vi "Drive Controller.vi"(8 "error in":errorcluster) -> ()   [LabVIEW 2018]
doc: "This VI executes continuously carrying out the current operation and responding to updates or new operation requests. It will often contain the timing or control code that is difficult to place directly in TeleOp. This VI generally opens all sensors and motors and isolates the rest of the robot code from knowing implementation details of how the operations are carried out."
uses:
  <vilib>/Rock Robotics/WPI/Framework/Completion Status.ctl
  Drive Setpoints.ctl
  Drive Operations.ctl
  <vilib>/Rock Robotics/WPI/SafetyOutput/WPI_SafetyOutputConfigMenu.ctl
  <vilib>/Rock Robotics/WPI/Utilities/WPI_GetSetVariantRefNum.vi
  <vilib>/Rock Robotics/SystemInterfaces/DIO/FPGA_DIOPWMChannel.ctl
  <vilib>/Rock Robotics/WPI/RobotDrive/WPI_RobotDriveOpen4MotorWithTalonSRX.vi
panel:
  in  "Interactive Values":T1
  in  "Buttons":cluster{"Execute Cmd":bool, "Abort Cmd":bool}
  out "Command Timing":cluster{"Start Time (ms)":u32, "Iterations":i32}
  out "Status":T3
  out "Setpoints":T4(graph)
  out "Current\nCmd":string
  # "Tip: The graph shows the motor setpoints. It may also be helpful to observe inputs and sensor values.\nYou may also want to display tuning or debugging controls."
  # "Interactive Command: You may fill in the settings for a command\nand schedule it with the Execute button. You can observe and abort\nany command while fine tuning the code for the controller."
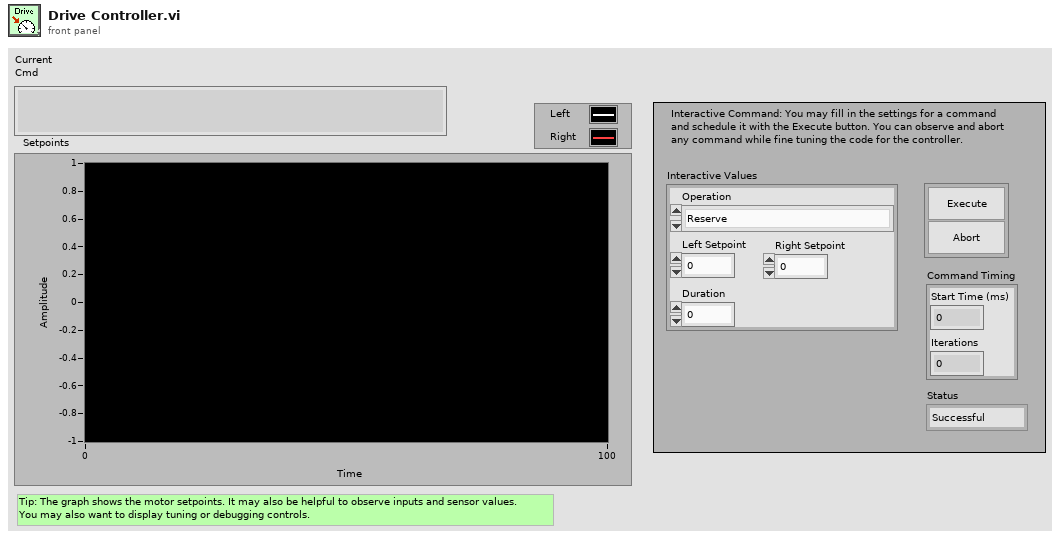
[diagram p1: front panel]
types:
  T1 = typedef "Drive Setpoints.ctl" = cluster{"Operation":T2, "Left Setpoint":dbl, "Right Setpoint":dbl, "Duration":dbl}
  T2 = typedef "Drive Operations.ctl" = enum16{"Reserve", "Read Current", "Immediate", "Drive for Time", "Drive for Distance"}
  T3 = typedef "Completion Status.ctl" = enum16{"Successful", "Aborted", "Incomplete"}
  T4 = cluster{"Left Setpoint":dbl, "Right Setpoint":dbl}
  T5 = typedef "WPI_SafetyOutputConfigMenu.ctl" = enum16{"Enable", "Disable"}
  T6 = typedef "FPGA_DIOPWMChannel.ctl" = enum8{"PWM 0", "PWM 1", "PWM 2", "PWM 3", "PWM 4", "PWM 5", "PWM 6", "PWM 7", "PWM 8", "PWM 9", "PWM MXP 0", "PWM MXP 1", "PWM MXP 2", "PWM MXP 3", "PWM MXP 4", "PWM MXP 5", "PWM MXP 6", "PWM MXP 7", "PWM MXP 8", "PWM MXP 9", "Invalid"}
  T7 = typedef "WPI_RobotDriveDevRef.ctl" = cluster{"DevStatus":errorcluster, "Motors[]":T8[], "Square Inputs":bool, "Max Output":dbl}
  T8 = typedef "WPI_MotorControlDeviceRef.ctl" = cluster{"DeviceStatus":errorcluster, "Type":T9, "PWM":cluster{"PWM Channel":T6, "DeadBand":T10}, "CAN":cluster{"Device Number":u8, "SetOutput VI Ref":variant, "GetOutput VI Ref":variant, "Enable VI Ref":variant, "Disable VI Ref":variant, "Data":variant}, "Invert":bool, "DIO PWM":cluster{"PWM \"Enable\" Channel":T6, "DIOChannel":T11, "PWM Rate":dbl}}
  T9 = typedef "WPI_MotorControlType.ctl" = enum16{"PWM", "CAN", "DIO PWM"}
  T10 = typedef "WPI_PWMDeadband.ctl" = cluster{"Name":string, "maxPositivePwm":i32, "minPositivePwm":i32, "centerPwm":i32, "maxNegativePwm":i32, "minNegativePwm":i32, "angularRange":u16}
  T11 = typedef "FPGA_DIOChannel.ctl" = enum8{"DIO 0", "DIO 1", "DIO 2", "DIO 3", "DIO 4", "DIO 5", "DIO 6", "DIO 7", "DIO 8", "DIO 9", "DIO MXP 0", "DIO MXP 1", "DIO MXP 2", "DIO MXP 3", "DIO MXP 4", "DIO MXP 5", "DIO MXP 6", "DIO MXP 7", "DIO MXP 8", "DIO MXP 9", "DIO MXP 10", "DIO MXP 11", "DIO MXP 12", "DIO MXP 13", "DIO MXP 14", "DIO MXP 15", "SPI Port CS1", "SPI Port CS2", "SPI Port CS3", "SPI Port MISO", "SPI Port MOSI", "Invalid"}
  T12 = typedef "Command Status Info.ctl" = cluster{"Name":string, "Status":T3, "notifier out":T13}
  T13 = typedef "Completion Notifier.ctl" = refnum<notifier>
  T14 = cluster{"SubSystem Data":T1, cluster{"Start Time (ms)":u32, "Iterations":i32}, cluster{"Command Info":T12, "Description":string, "Default Command":T1, "queue out":refnum<queue>, "Subsystem Name":string}}
  T15 = cluster{"SubSystem Data":T1, cluster{"Start Time (ms)":u32, "Iterations":i32}, "Default Command Arguments":cluster{"Command Info":T12, "Description":string, "Default Command":T1, "queue out":refnum<queue>, "Subsystem Name":string}}
  T16 = cluster{"Don't move motors while reserved":dbl, "Don't move motors while reserved":dbl}
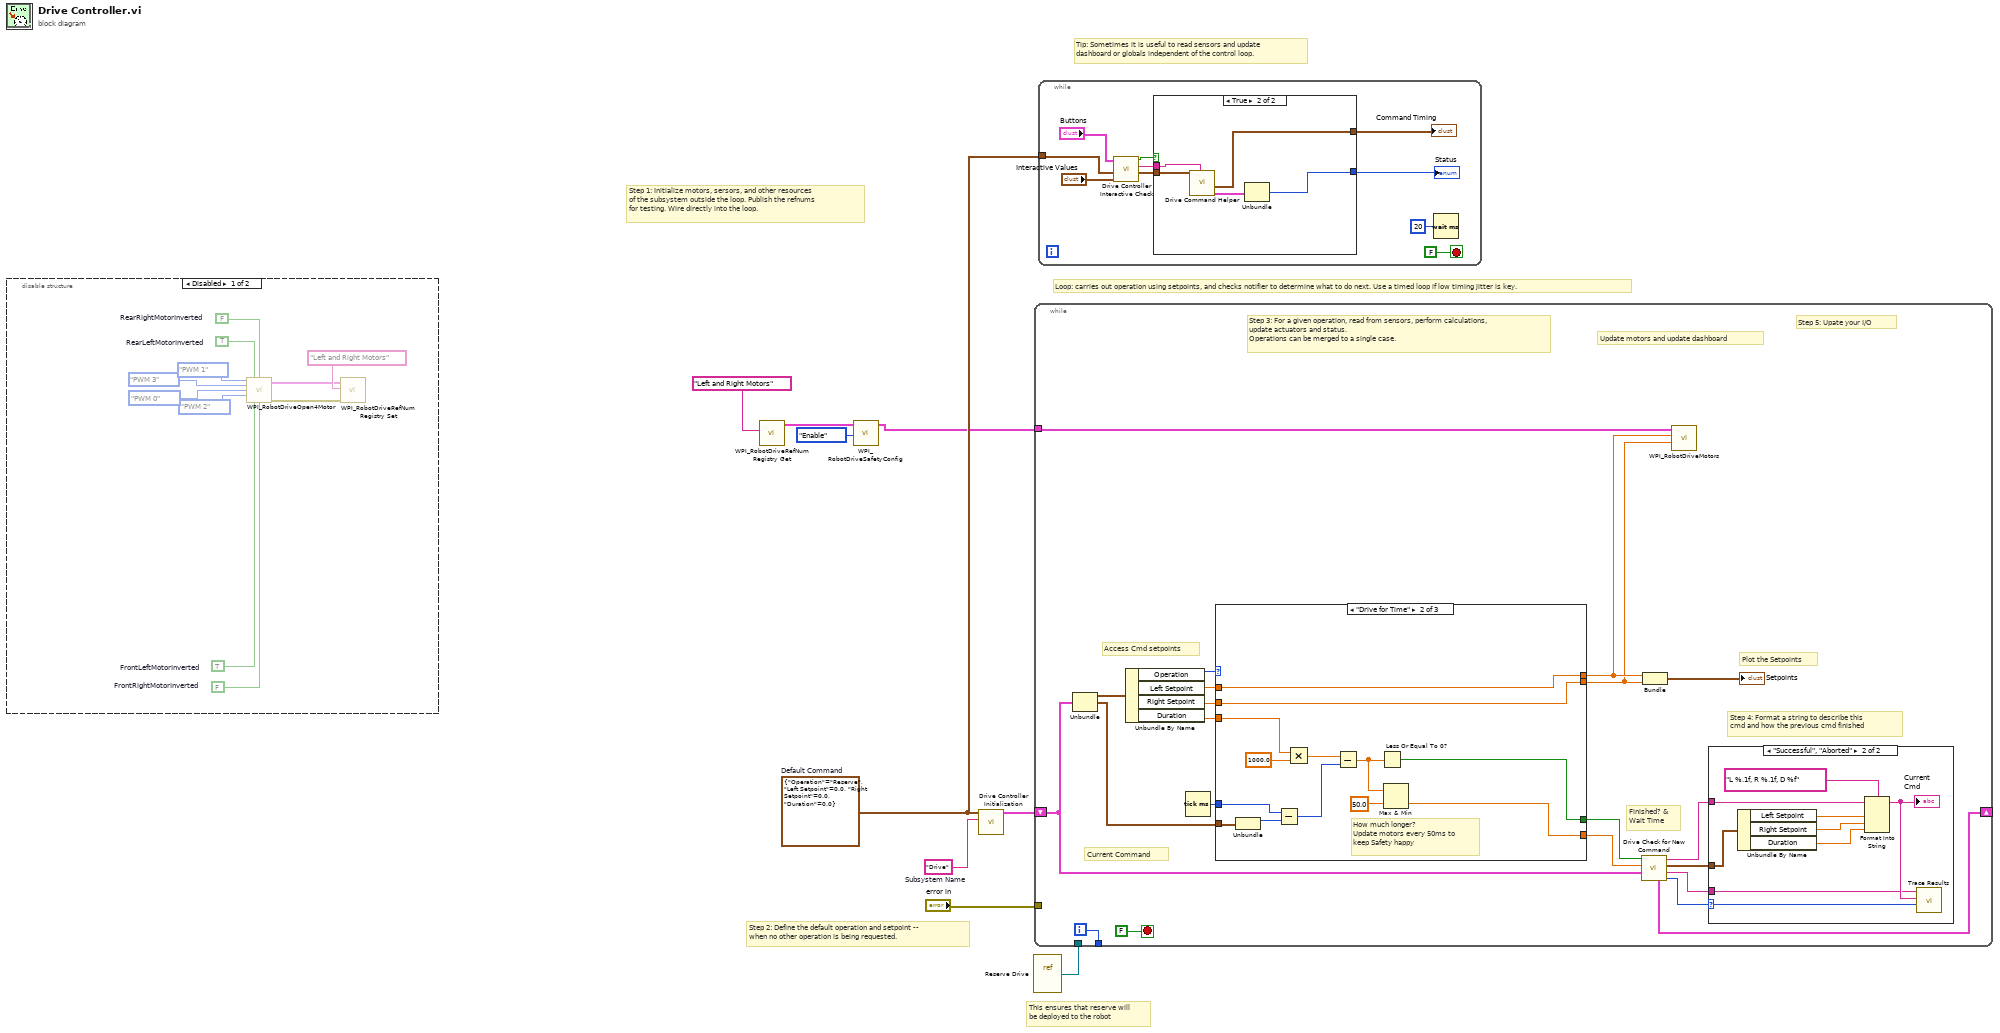
[diagram p0: block diagram]
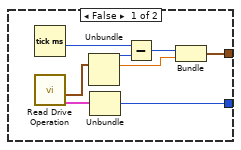
[diagram p3: hidden frame]
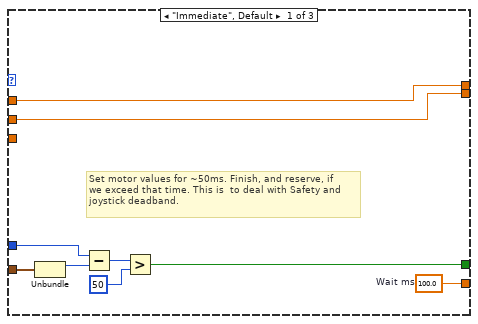
[diagram p5: hidden frame]
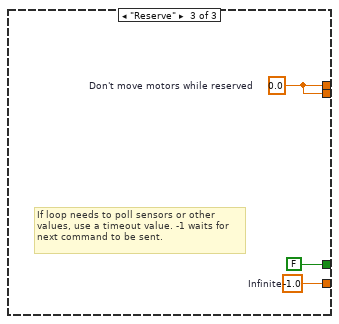
[diagram p6: hidden frame]
diagram:
  w5 = T1 {"Operation"=enum."Reserve", "Left Setpoint"=0.0, "Right Setpoint"=0.0, "Duration"=0.0}  # Default Command
  w9 = "Drive"  # Subsystem Name
  # "This ensures that reserve will\nbe deployed to the robot"
  # "Tip: Sometimes it is useful to read sensors and update\ndashboard or globals independent of the control loop."
  # "Step 2: Define the default operation and setpoint --\nwhen no other operation is being requested."
  # "Step 1: Initialize motors, sersors, and other resources\nof the subsystem outside the loop. Publish the refnums\nfor testing. Wire directly into the loop."
  # "Loop: carries out operation using setpoints, and checks notifier to determine what to do next. Use a timed loop if low timing jitter is key."
  n1 = disable-structure shown="Disabled" {
    frame Disabled {
      w19 = TRUE  # FrontLeftMotorInverted
      w16 = FALSE  # FrontRightMotorInverted
      w18 = TRUE  # RearLeftMotorInverted
      w17 = FALSE  # RearRightMotorInverted
      n2 = call-poly <vilib>:"WPI_RobotDriveOpen4Motor.vi"("Rear Left Motor"=FPGA_DIOPWMChannel."PWM 1" ("Rear Right Motor"), "Rear Left Motor Inverted"=w18, "Rear Right Motor Inverted"=w17, "Rear Right Motor"=FPGA_DIOPWMChannel."PWM 3" ("Front Left Motor"), "Front Left Motor"=FPGA_DIOPWMChannel."PWM 0" ("Rear Left Motor"), "Front Right Motor"=FPGA_DIOPWMChannel."PWM 2", "Front Left Motor Inverted"=w19, "Front Right Motor Inverted"=w16) -> ("RobotDriveDevRef"=w12:T7, "error out"=w11:errorcluster)  [unwired: 6 in]
      n3 = call <vilib>:"WPI_RobotDriveRefNum Registry Set.vi"("error in (no error)"=w11, "refnum name"="Left and Right Motors", "RobotDriveDevRef"=w12) -> ()  [unwired: 1 in, 8 out]
    }
    frame Enabled {
    }
  }
  n4 = call <vilib>:"WPI_RobotDriveRefNum Registry Get.vi"("refnum name"="Left and Right Motors") -> ("RobotDriveDevRef"=w4:T7)  [unwired: 9 in, 1 out]
  n5 = call <vilib>:"WPI_RobotDriveSafetyConfig.vi"("mode"=WPI_SafetyOutputConfigMenu."Enable", "RobotDriveDevRef"=w4) -> ("RobotDriveDevRef"=w1:T7)  [unwired: 8 in, 1 out]
  n6 = call "Drive Controller Initialization.vi"("Subsystem Name"=w9, "Default Command"=w5) -> ("Current Command"=w7:T14)  [unwired: 9 in]
  n7 = vi-ref "Reserve Drive.vi"() -> (w6:refnum<vi>)
  n8 = while {
    shift-right: [w31] -> _
    shift-left: w7 -> [w24]
    tunnel: [w40] -> _
    tunnel: "error in" -> [_]
    tunnel: w6 -> [_]
    tunnel: w1 -> [w23]
    i -> [w40]
    stop <- FALSE stop-if-true
    # "Step 5: Upate your I/O"
    # "Step 4: Format a string to describe this\ncmd and how the previous cmd finished"
    # "Current Command"
    # "Update motors and update dashboard"
    # "Plot the Setpoints"
    # "Access Cmd setpoints"
    # "Finished? &\nWait Time"
    # "Step 3: For a given operation, read from sensors, perform calculations,\nupdate actuators and status.\nOperations can be merged to a single case."
    n9 = Unbundle(w24) -> ("SubSystem Data"=w38:T1, w25:cluster{"Start Time (ms)":u32, "Iterations":i32})  [unwired: 1 out]
    n10 = Unbundle By Name(w38) -> ("Operation"=w37:T2, "Left Setpoint"=w36:dbl, "Right Setpoint"=w35:dbl, "Duration"=w34:dbl)
    n11 = Tick Count (ms)() -> (millisecond timer value=w33:u32)
    n12 = case shown="\"Drive for Time\"" w37 {
      tunnel: [w59 w60 w75] -> w30
      tunnel: [w52 w67 FALSE ("ignore previous (F)")] -> w29
      tunnel: w25 -> [w51 w69 _]
      tunnel: [w58 w66 w73] -> w22
      tunnel: [w57 w65 w73] -> w21
      tunnel: w36 -> [w58 w66 _]
      tunnel: w35 -> [w57 w65 _]
      tunnel: w34 -> [_ w64 _]
      tunnel: w33 -> [w53 w63 _]
      frame "Immediate", Default {
        w59 = 100.0  # Wait ms
        # "Set motor values for ~50ms. Finish, and reserve, if\nwe exceed that time. This is  to deal with Safety and\njoystick deadband."
        n13 = Unbundle(w51) -> ("Start Time (ms)"=w54:u32)  [unwired: 1 out]
        n14 = Subtract(x=w53, y=w54) -> (x-y=w55:u32)
        n15 = Greater?(x=w55, y=u8 50 ("Left Motor")) -> (0:w52:bool)
      }
      frame "Drive for Time" {
        # "How much longer?\nUpdate motors every 50ms to\nkeep Safety happy"
        n16 = Unbundle(w69) -> ("Start Time (ms)"=w68:u32)  [unwired: 1 out]
        n17 = Subtract(x=w63, y=w68) -> (x-y=w72:u32)
        n18 = Multiply(x=w64, y=1000.0) -> (x*y=w71:dbl)
        n19 = Subtract(x=w71, y=w72) -> (x-y=w62:dbl)
        n20 = Less Or Equal To 0?(x=w62) -> (x <= 0?=w67:bool)
        n21 = Max & Min(x=w62, y=50.0) -> (min(x,y)=w60:dbl)  [unwired: 1 out]
      }
      frame "Reserve" {
        w73 = 0.0  # Don't move motors while reserved
        w75 = -1.0  # Infinite
        # "If loop needs to poll sensors or other\nvalues, use a timeout value. -1 waits for\nnext command to be sent."
      }
    }
    n22 = call "Drive Check for New Command.vi"("input cluster"=w24, "Wait time (ms)"=w30, "Finished?"=w29) -> ("Completion"=w32:T3, "Subsystem Name"=w26:string, "Current Command"=w27:T1, "Initial Trace String"=w28:string, "Next Command"=w31:T15)  [unwired: 4 in]
    n23 = Bundle("Don't move motors while reserved"=w22, "Don't move motors while reserved"=w21) -> (→"Setpoints":T16)  [unwired: 1 in]
    n24 = call <vilib>:"WPI_RobotDriveMotors.vi"("RightSpeed"=w21, "LeftSpeed"=w22, "RobotDriveDevRef"=w23) -> ()  [unwired: 6 in, 3 out]
    n25 = case shown="\"Successful\", \"Aborted\"" w32 {
      selector: w32 -> [_ w50]
      tunnel: w28 -> [_ w45]
      tunnel: w27 -> [_ w46]
      tunnel: w26 -> [_ w42]
      frame "Incomplete", Default {
        # "Continuing current command"
      }
      frame "Successful", "Aborted" {
        # "Report and setup for next command"
        n26 = Unbundle By Name(w46) -> ("Left Setpoint"=w48:dbl, "Right Setpoint"=w49:dbl, "Duration"=w43:dbl)
        n27 = Format Into String(format string="L %.1f, R %.1f, D %f", initial string=w45, w48, w49, w43) -> (resulting string=w44:string)  [unwired: 1 in, 1 out]
        "Current\nCmd" <- w44
        n28 = call <vilib>:"Trace Results.vi"("Status of previous command"=w50, "Description"=w44, "Subsystem"=w42) -> ()  [unwired: 9 in]
      }
    }
  }
  n29 = while {
    tunnel: w5 -> [w77]
    stop <- FALSE stop-if-true
    n30 = call "Drive Controller Interactive Check.vi"("Interactive Command In"="Interactive Values", "Default Command"=w77, "Buttons"="Buttons") -> ("Interactive Command Out"=w79:T1, "Trace String"=w80:string, "Schedule"=w81:bool)  [unwired: 6 in]
    n31 = case shown="True" w81 {
      tunnel: [w90 w98] -> w82
      tunnel: [w89 w95] -> w83
      tunnel: w80 -> [_ w94]
      tunnel: w79 -> [_ w96]
      frame False {
        n32 = Tick Count (ms)() -> (millisecond timer value=w93:u32)
        n33 = call "Read Drive Operation.vi"() -> ("Command Info"=w87:T12, "SubSystem Data"=w86:T1)  [unwired: 9 in, 1 out]
        n34 = Unbundle(w86) -> ("Operation"=w91:T2, "Left Setpoint"=w88:dbl)  [unwired: 2 out]
        n35 = Unbundle(w87) -> ("Status"=w90:T3)  [unwired: 2 out]
        n36 = Subtract(x=w93, y=w91) -> (x-y=w92:u32)
        n37 = Bundle(w92, "Left Setpoint"=w88) -> (w89:cluster{u32, "Left Setpoint":dbl})  [unwired: 1 in]
      }
      frame True {
        n38 = call "Drive Command Helper.vi"("Description"=w94, "SubSystem Data"=w96) -> ("Command Info Out"=w97:T12, "Command Timing"=w95:cluster{"Start Time (ms)":u32, "Iterations":i32})  [unwired: 7 in, 1 out]
        n39 = Unbundle(w97) -> ("Status"=w98:T3)  [unwired: 2 out]
      }
    }
    "Status" <- w82
    "Command Timing" <- w83
    n40 = Wait (ms)(milliseconds to wait=u32 20) -> ()  [unwired: 1 out]
  }
